vi "Experiment 3.vi"() -> ()   [LabVIEW 2026]
doc: "Experiment 3"
uses:
  <vilib>/Analysis/baseanly.llb/Mean (DBL).vi
  <vilib>/Analysis/NI_AALBase.lvlib
panel:
  out "Execution Time - Per Call (us)":dbl format="%.6f"
  out "Execution Time - 1M Calls (seconds)":dbl format="%.6f"
  out "Output":dbl[](array[numeric]) format="%.3f"
  # "Experiment 3"
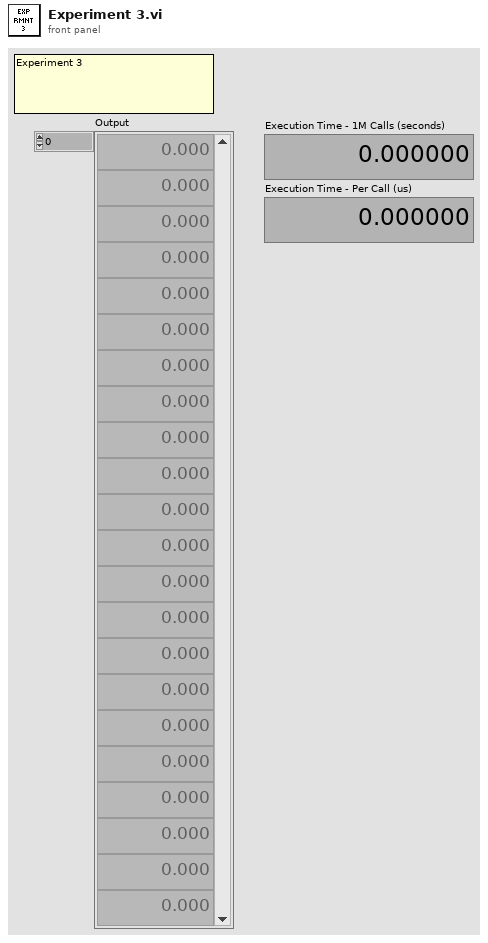
[diagram p1: front panel]
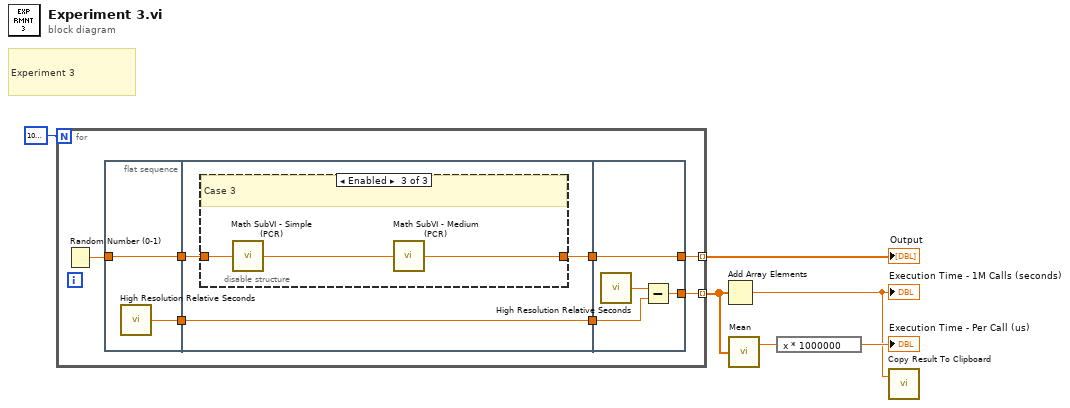
[diagram p0: block diagram]
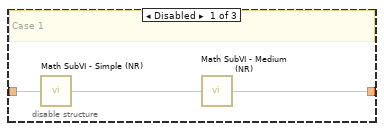
[diagram p2: hidden frame]
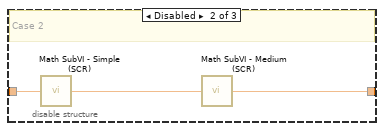
[diagram p3: hidden frame]
diagram:
  # "Experiment 3"
  n1 = for {
    N: 1000000 -> [_]
    tunnel: [w13] -> w6 mode=indexing
    tunnel: [w7] -> w4 mode=indexing
    n2 = Random Number (0-1)() -> (number: 0 to 1=w12:dbl)
    n3 = flat-sequence {
      tunnel: w12 -> [w15]
      tunnel: [w15] -> w11
      tunnel: [w14] -> w8
      tunnel: w11 -> [w16]
      tunnel: [w17] -> w10
      tunnel: [w18] -> w9
      tunnel: w8 -> [w18]
      tunnel: [w31] -> w13
      tunnel: w10 -> [w31]
      tunnel: w9 -> [w29]
      tunnel: [w28] -> w7
      frame #0 {
        n4 = call <vilib>:"High Resolution Relative Seconds.vi"() -> ("relative seconds"=w14:dbl)
      }
      frame #1 {
        n5 = disable-structure shown="Enabled" {
          disable-tunnel: [w19 w22 w25] -> w17
          disable-tunnel: w16 -> [w20 w23 w26]
          frame Disabled {
            # "Case 1"
            n6 = call "Math SubVI - Simple (NR).vi"("Input"=w20) -> ("Output"=w21:dbl)
            n7 = call "Math SubVI - Medium (NR).vi"("Input"=w21) -> ("Output"=w19:dbl)
          }
          frame Disabled {
            # "Case 2"
            n8 = call "Math SubVI - Simple (SCR).vi"("Input"=w23) -> ("Output"=w24:dbl)
            n9 = call "Math SubVI - Medium (SCR).vi"("Input"=w24) -> ("Output"=w22:dbl)
          }
          frame Enabled {
            # "Case 3"
            n10 = call "Math SubVI - Simple (PCR).vi"("Input"=w26) -> ("Output"=w27:dbl)
            n11 = call "Math SubVI - Medium (PCR).vi"("Input"=w27) -> ("Output"=w25:dbl)
          }
        }
      }
      frame #2 {
        n12 = call <vilib>:"High Resolution Relative Seconds.vi"() -> ("relative seconds"=w30:dbl)
        n13 = Subtract(x=w30, y=w29) -> (x-y=w28:dbl)
      }
    }
  }
  "Output" <- w6
  n14 = Add Array Elements(numeric array=w4) -> (sum=w1:dbl)
  "Execution Time - 1M Calls (seconds)" <- w1
  n15 = call-poly <vilib>:"Mean.vi"("X"=w4) -> ("mean"=w3:dbl)  [unwired: 1 out]
  n16 = expression code="x * 1000000"(w3) -> (→"Execution Time - Per Call (us)":dbl)
  n17 = call "Copy Result To Clipboard.vi"("Input"=w1) -> ()  [unwired: 1 in]
